vi "SVL Send Data to Waterfall (Array of Spectra).vi"(0 "waterfall ref":refnum<vi>, 1 "axis labels":T1, 5 "waterfall data":cluster{"f0":dbl, "df":dbl, "magnitude":dbl[]}[](array[cluster]) {"magnitude" format="%.2p"; "df" format="%.2p"; "f0" format="%.2p"}, 9 "y0 and delta y":cluster{"y0":dbl, "delta y":dbl}={"y0"=0.0, "delta y"=1.0} {"delta y" format="%.2f"; "y0" format="%.2f"}, 11 "error in (no error)":errorcluster, 12 "settings":T2={"clear graph before redrawing (F)"=FALSE, "set baseline (F)"=FALSE, "baseline"=0.0, "autoscale (T)"=TRUE} {"baseline" format="%.2f"}, 13 "frontmost (T)":bool=TRUE) -> (4 "dup waterfall ref":refnum<vi>, 15 "error out":errorcluster)   [LabVIEW 2017]
doc: "Sends the waterfall data to the waterfall display. You can use this polymorphic VI to send waterfall data to the waterfall display using a 2D array or a cluster. The data type you wire to the <B>waterfall data</B> input determines the polymorphic instance to use."
uses:
  <vilib>/addons/Sound and Vibration/compatibility/Waterfall/subVIs/svl_Waterfall Global.vi
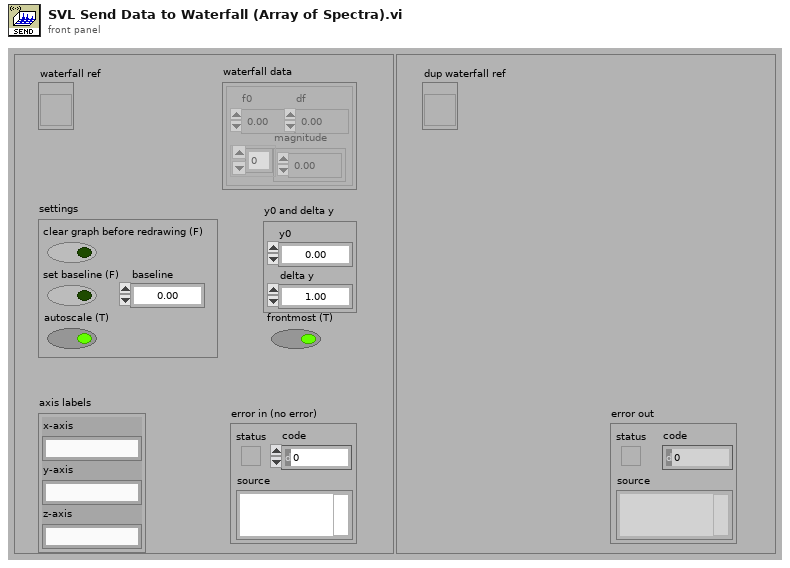
[diagram p1: front panel]
types:
  T1 = cluster{"x-axis":string, "y-axis":string, "z-axis":string}
  T2 = cluster{"clear graph before redrawing (F)":bool, "set baseline (F)":bool, "baseline":dbl, "autoscale (T)":bool}
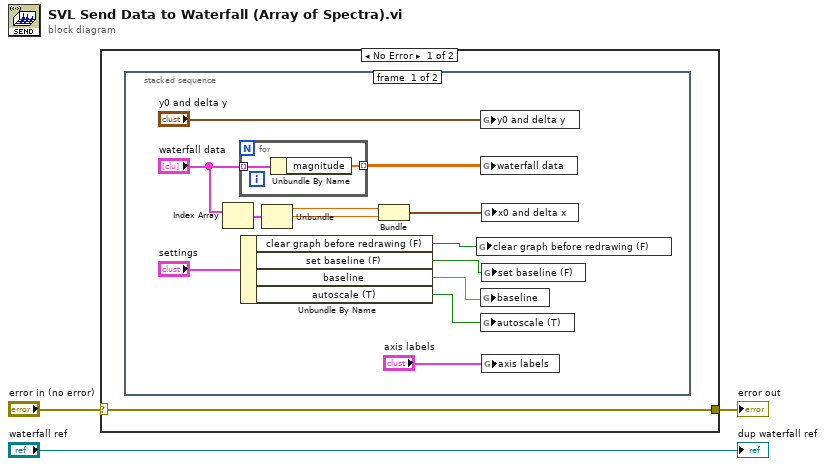
[diagram p0: block diagram]
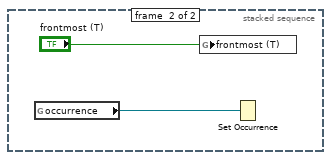
[diagram p2: hidden frame]
diagram:
  n1 = case shown="No Error" "error in (no error)" {
    selector: "error in (no error)" -> [w4 w22]
    tunnel: [w4 w22] -> w1
    frame No Error {
      n2 = stacked-sequence {
        frame #0 {
          n3 = Index Array(array="waterfall data") -> (element=w9:cluster{"f0":dbl, "df":dbl, "magnitude":dbl[]})  [unwired: 1 in]
          n4 = for {
            tunnel: "waterfall data" -> [w19] mode=indexing
            tunnel: [w18] -> w11 mode=indexing
            n5 = Unbundle By Name(w19) -> ("magnitude"=w18:dbl[])
          }
          n6 = Unbundle By Name("settings") -> ("clear graph before redrawing (F)"=w15:bool, "set baseline (F)"=w14:bool, "baseline"=w13:dbl, "autoscale (T)"=w12:bool)
          n7 = Unbundle(w9) -> ("f0"=w8:dbl, "df"=w7:dbl)  [unwired: 1 out]
          n8 = Bundle("f0"=w8, "df"=w7) -> (w6:cluster{"f0":dbl, "df":dbl})  [unwired: 1 in]
          n9 = global write "svl_Waterfall Global.vi" "clear graph before redrawing (F)"(w15) -> ()
          n10 = global write "svl_Waterfall Global.vi" "y0 and delta y"("y0 and delta y") -> ()
          n11 = global write "svl_Waterfall Global.vi" "waterfall data"(w11) -> ()
          n12 = global write "svl_Waterfall Global.vi" "baseline"(w13) -> ()
          n13 = global write "svl_Waterfall Global.vi" "autoscale (T)"(w12) -> ()
          n14 = global write "svl_Waterfall Global.vi" "x0 and delta x"(w6) -> ()
          n15 = global write "svl_Waterfall Global.vi" "set baseline (F)"(w14) -> ()
          n16 = global write "svl_Waterfall Global.vi" "axis labels"("axis labels") -> ()
        }
        frame #1 {
          n17 = global read "svl_Waterfall Global.vi" "occurrence"() -> (w20:refnum<k4>)
          n18 = global write "svl_Waterfall Global.vi" "frontmost (T)"("frontmost (T)") -> ()
          n19 = Set Occurrence(w20) -> ()
        }
      }
    }
    frame Error {
    }
  }
  "error out" <- w1
  "dup waterfall ref" <- "waterfall ref"
